vi "Process Packet from Server.vi"(8 "error in (no error)":errorcluster, 10 "Incoming Packet":refnum<class "ControlPacket.lvclass">, 11 "Session in":refnum<class "Session.lvclass">) -> (0 "error out":errorcluster, 3 "Session out":refnum<class "Session.lvclass">)   [LabVIEW 2013, in "MQTT Server.lvlib" / "Session.lvclass"]
uses:
  Session.lvclass
  Control Packets/ControlPacket/ControlPacket.lvclass
  MQTT_Base/Request -- cluster.ctl
  MQTT_Base/Response -- cluster.ctl
  Control Packets/ControlPacket/ControlPacket.lvclass/ControlPacket.ctl
  Session.lvclass/Session.ctl
  Read SessionState.vi
  MQTT_Base/MQTT_Base.lvclass
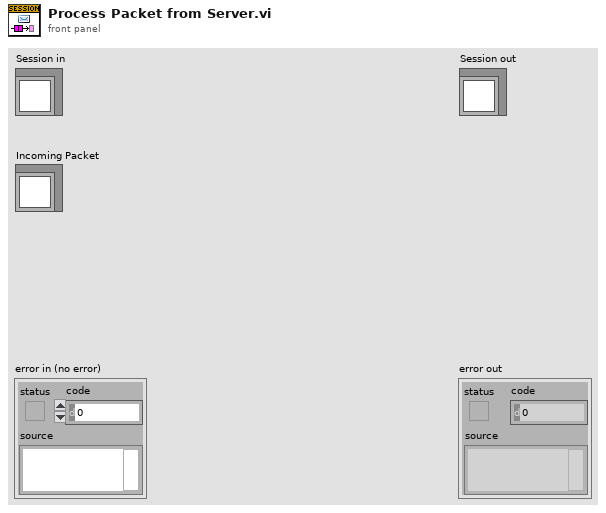
[diagram p1: front panel]
types:
  T1 = typedef "MQTT Server.lvlib/MQTT_Base.lvclass/Request -- cluster.ctl" = cluster{"Packet":refnum<class "ControlPacket.lvclass">, "SessionMailbox":refnum<queue>}
  T2 = typedef "MQTT Server.lvlib/Session.lvclass/Pending ACKs -- cluster.ctl" = cluster{"Message":refnum<class "ControlPacket.lvclass">, "[ACK]":refnum<notifier>[], "Packet Identifier":u16}
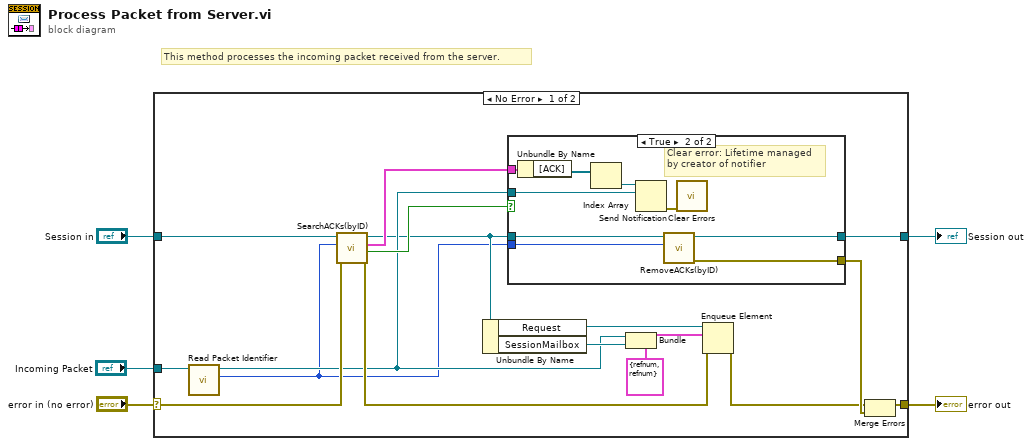
[diagram p0: block diagram]
diagram:
  # "This method processes the incoming packet received from the server."
  n1 = case shown="No Error" "error in (no error)" {
    selector: "error in (no error)" -> [w16 w34]
    tunnel: [w8 w34] -> w4
    tunnel: [w11 w33] -> w2
    tunnel: "Session in" -> [w18 w33]
    tunnel: "Incoming Packet" -> [w6 _]
    frame No Error {
      n2 = call "Read Packet Identifier.vi"("ControlPacket in"=w6) -> ("Packet Identifier"=w7:u16, "ControlPacket out"=w13:refnum<class "ControlPacket.lvclass">)  [unwired: 9 in]
      n3 = call "SearchACKs(byID).vi"("error in (no error)"=w16, "Packet Identifier"=w7, "Session in"=w18) -> ("error out"=w17:errorcluster, "found?"=w15:bool, "Pending ACK"=w14:T2, "Session out"=w12:refnum<class "Session.lvclass">)  [unwired: 5 in]
      n4 = Unbundle By Name(w12) -> ("Request"=w22:refnum<queue>, "SessionMailbox"=w21:refnum<queue>)
      n5 = case shown="True" w15 {
        tunnel: w14 -> [_ w32]
        tunnel: w13 -> [_ w29]
        tunnel: w12 -> [w23 w27]
        tunnel: [w23 w26] -> w11
        tunnel: [_ w24] -> w10
        tunnel: w7 -> [_ w25]
        frame False {
        }
        frame True {
          # "Clear error: Lifetime managed\nby creator of notifier"
          n6 = Unbundle By Name(w32) -> ("[ACK]"=w31:refnum<notifier>[])
          n7 = Index Array(array=w31) -> (element=w30:refnum<notifier>)  [unwired: 1 in]
          n8 = Send Notification(notification=w29, notifier=w30) -> (error out=w28:errorcluster)  [unwired: 1 in, 1 out]
          n9 = call "RemoveACKs(byID).vi"("Packet Identifier"=w25, "Session in"=w27) -> ("error out"=w24:errorcluster, "Session out"=w26:refnum<class "Session.lvclass">)  [unwired: 8 in]
          n10 = call <vilib>:"Clear Errors.vi"("error in (no error)"=w28) -> ()  [unwired: 6 in, 1 out]
        }
      }
      n11 = Bundle(cluster=T1 {"Packet"=refnum, "SessionMailbox"=refnum} ("Request"), "Packet"=w13, "SessionMailbox"=w21) -> (w20:T1)
      n12 = Enqueue Element(queue=w22, element=w20, error in (no error)=w17) -> (error out=w9:errorcluster)  [unwired: 1 in, 2 out]
      n13 = Merge Errors(w9, w10) -> (w8:errorcluster)
    }
    frame Error {
    }
  }
  "error out" <- w4
  "Session out" <- w2
